vi "Send TDMS Cleanup.vi"(1 "Auto Clust":T1={"Automate?"=FALSE, "Num Parabs"=1, "Patterns Array"=[], "Phase Array"=[]} {"Num Parabs" min=1 step=1}, 2 "Movement?":bool, 4 "Task info":T2={"Number of Trials"=1, "Sampling Rate (Hz)"=200, "Trial Duration (s)"=10, "Adjusted MVC (N)"=5.0, "R Phase"=0, "L Phase"=0, "L Pattern"=1, "R Pattern"=1, "Time Between Trials (s)"=5, "Lissajous Speed"=200} {"Lissajous Speed" min=1 max=200; "Time Between Trials (s)" min=1 step=1; "R Pattern" min=1 max=20 step=1; "L Pattern" min=1 max=20 step=1; "L Phase" min=-180 max=180 step=1; "R Phase" min=-180 max=180 step=1; "Adjusted MVC (N)" min=1.0 max=50.0 step=0.10000000149011612; "Trial Duration (s)" min=1 step=1; "Sampling Rate (Hz)" min=1 step=1; "Number of Trials" min=1 step=1}, 5 "Force TDMS File":refnum<k34>, 6 "Task Selection":T3={"Task Type Select"=enum."Frequency Task", "Input Select Type"=enum."Force Input", "Collect EMG?"=FALSE, "Collect acceleration?"=FALSE, "EMG Rate"=200, "Acceleration Rate"=200} {"Acceleration Rate" min=1 step=1; "EMG Rate" min=1 step=1}, 7 "Priority":T4=enum."Normal" caption="Message Priority (Normal)", 8 "error in (no error)":errorcluster, 9 "Accel TDMS File":refnum<k34>, 10 "TDMS File":path, 11 "Message Enqueuer in":refnum<class "Message Enqueuer.lvclass">) -> (0 "error out":errorcluster, 3 "Message Enqueuer out":refnum<class "Message Enqueuer.lvclass">)   [LabVIEW 2020, in "Logging.lvlib" / "TDMS Cleanup Msg.lvclass"]
doc: "Sends the <b>Logging.lvlib:TDMS Cleanup Msg.lvclass</b> message.\n\nThis message will call <b>TDMS Cleanup.vi</b> on the <b>Logging.lvlib:Logging.lvclass</b> actor.\n\n<b>TDMS Cleanup.vi Description</b>"
uses:
  TDMS Cleanup Msg.lvclass
  <vilib>/ActorFramework/Message Enqueuer/Message Enqueuer.lvclass
  <vilib>/ActorFramework/Message Enqueuer/Message Priority.ctl
  Task selection df.ctl
  Task info df.ctl
  Automate df.ctl
  C:/Program Files/National Instruments/LabVIEW 2020/vi.lib/ActorFramework/Message/Message.lvclass
  TDMS Cleanup Msg.lvclass/TDMS Cleanup Msg.ctl
  <vilib>/ActorFramework/Message Enqueuer/Message Enqueuer.lvclass/Message Enqueuer.ctl
  <vilib>/ActorFramework/Message Priority Queue/Priority Enqueue.vi
panel:
  # "Patterns"
  # "Phase"
  # "Left        Right"
  # "Left        Right"
  # "Left Arm"
  # "Right Arm"
  # "Input Type"
  # "Task Type"
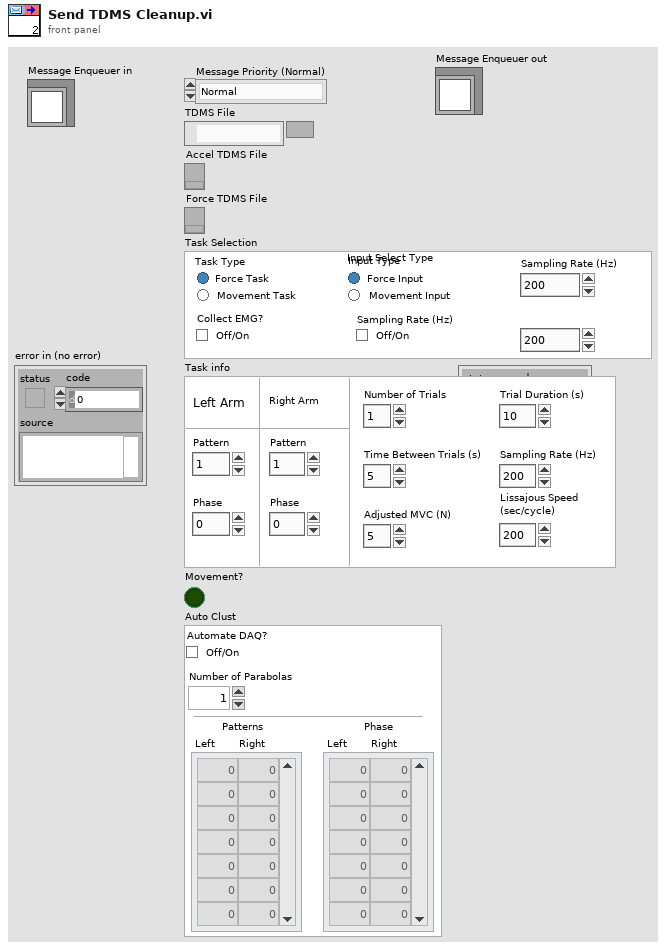
[diagram p1: front panel]
types:
  T1 = typedef "Automate df.ctl" = cluster{"Automate?":bool, "Num Parabs":u16, "Patterns Array":u8[][], "Phase Array":i32[][]}
  T2 = typedef "Task info df.ctl" = cluster{"Number of Trials":u8, "Sampling Rate (Hz)":u16, "Trial Duration (s)":u8, "Adjusted MVC (N)":dbl, "R Phase":i32, "L Phase":i32, "L Pattern":u8, "R Pattern":u8, "Time Between Trials (s)":u8, "Lissajous Speed":u16}
  T3 = typedef "Task selection df.ctl" = cluster{"Task Type Select":enum32{"Frequency Task", "Scanning Task"}, "Input Select Type":enum32{"Force Input", "Movement Input"}, "Collect EMG?":bool, "Collect acceleration?":bool, "EMG Rate":u16, "Acceleration Rate":u16}
  T4 = typedef "Actor Framework.lvlib/Message Enqueuer.lvclass/Message Priority.ctl" = enum16{"Low", "Normal", "High"}
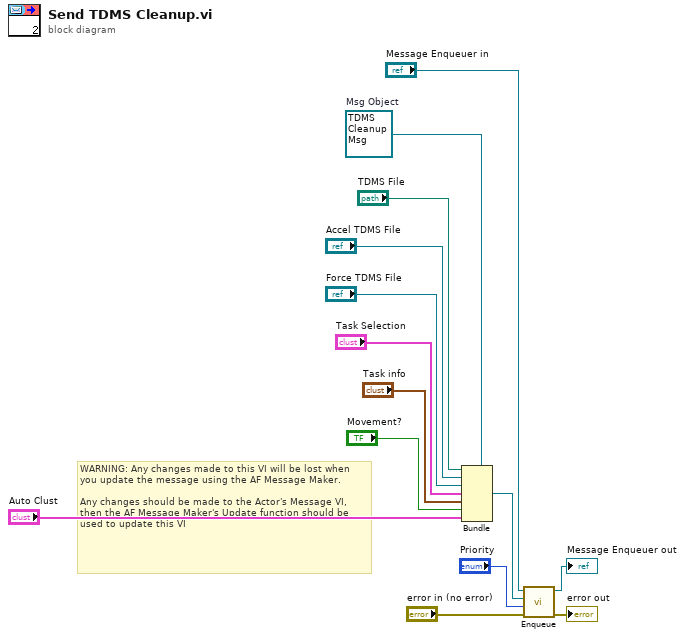
[diagram p0: block diagram]
diagram:
  w7 = refnum<class "TDMS Cleanup Msg.lvclass"> refnum  # Msg Object
  # "WARNING: Any changes made to this VI will be lost when you update the message using the AF Message Maker.\n\nAny changes should be made to the Actor's Message VI, then the AF Message Maker's Update function should be used to update this VI"
  n1 = Bundle(cluster=w7, "TDMS File", "Accel TDMS File", "Force TDMS File", "Task Selection", "Task info", "Movement?", "Auto Clust") -> (w2:refnum<class "TDMS Cleanup Msg.lvclass">)
  n2 = call <vilib>:"Enqueue.vi"("error in (no error)"="error in (no error)", "Message Priority (Normal)"="Priority", "Message"=w2, "Message Enqueuer in"="Message Enqueuer in") -> ("error out"=→"error out":errorcluster, "Message Enqueuer out"=→"Message Enqueuer out":refnum<class "Message Enqueuer.lvclass">)  [unwired: 6 in]
